vi "xwav2x.vi"(4 "xwave":T1={"attributes"=variant, "X"={"start"=0.0, "delta"=0.0, "units"="index", "dim"="au"}, "Y"={"data"=[], "units"="au"}}) -> (1 "X":dbl[](array[numeric]))   [LabVIEW 2015]
uses:
  xwav.ctl
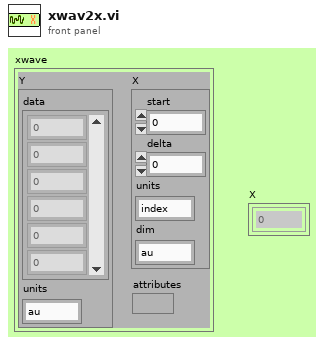
[diagram p1: front panel]
types:
  T1 = typedef "xwav.ctl" = cluster{"attributes":variant, "X":cluster{"start":dbl, "delta":dbl, "units":string, "dim":string}, "Y":cluster{"data":dbl[], "units":string}}
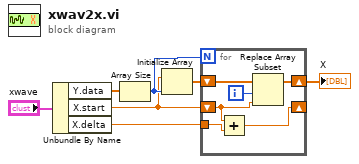
[diagram p0: block diagram]
diagram:
  n1 = Unbundle By Name("xwave") -> ("Y.data"=w2:dbl[], "X.start"=w4:dbl, "X.delta"=w3:dbl)
  n2 = Array Size(array=w2) -> (size(s)=w6:i32)
  n3 = Initialize Array(w4, w6) -> (w5:dbl[])
  n4 = for {
    N: w6 -> [_]
    shift-right: [w12] -> w1
    shift-left: w5 -> [w13]
    shift-right: [w8] -> _
    shift-left: w4 -> [w9]
    tunnel: w3 -> [w10]
    i -> [w11]
    n5 = Add(x=w9, y=w10) -> (x+y=w8:dbl)
    n6 = Replace Array Subset(array=w13, new element=w9, index=w11) -> (w12:dbl[])
  }
  "X" <- w1
